vi "RichToFlatni_measurementlink_sessionmanagement_v1_MultiplexerSessionInformation.vi"(5 "OutputClusterType":T1, 11 "InputCluster":T3) -> (3 "OutputCluster":T1)   [LabVIEW 2020, in "MeasurementLink Session Management Client.lvlib"]
uses:
  MeasurementLink Session Management Client.lvlib
  ni_measurementlink_sessionmanagement_v1_MultiplexerSessionInformation.ctl
  nidevice_grpc_Session.ctl
  ni_measurementlink_sessionmanagement_v1_MultiplexerSessionInformation_Flat.ctl
  nidevice_grpc_Session_Flat.ctl
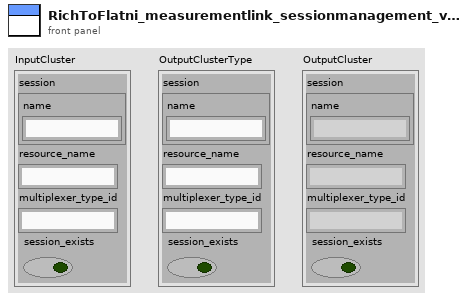
[diagram p1: front panel]
types:
  T1 = typedef "MeasurementLink Session Management Client.lvlib/ni_measurementlink_sessionmanagement_v1_MultiplexerSessionInformation_Flat.ctl" = cluster{"session":T2, "resource_name":string, "multiplexer_type_id":string, "session_exists":bool}
  T2 = typedef "MeasurementLink Session Management Client.lvlib/nidevice_grpc_Session_Flat.ctl" = cluster{"name":string}
  T3 = typedef "MeasurementLink Session Management Client.lvlib/ni_measurementlink_sessionmanagement_v1_MultiplexerSessionInformation.ctl" = cluster{"session":T4, "resource_name":string, "multiplexer_type_id":string, "session_exists":bool}
  T4 = typedef "MeasurementLink Session Management Client.lvlib/nidevice_grpc_Session.ctl" = cluster{"name":string}
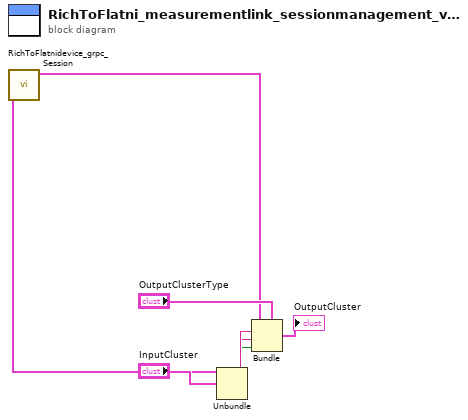
[diagram p0: block diagram]
diagram:
  n1 = Unbundle "Unbundle"("InputCluster") -> ("session"=w5:T4, "resource_name"=w3:string, "multiplexer_type_id"=w2:string, "session_exists"=w1:bool)
  n2 = call "RichToFlatnidevice_grpc_Session.vi"("InputCluster"=w5) -> ("OutputCluster"=w4:T2)  [unwired: 10 in]
  n3 = Bundle "Bundle"(cluster="OutputClusterType", "session"=w4, "resource_name"=w3, "multiplexer_type_id"=w2, "session_exists"=w1) -> (→"OutputCluster":T1)
